vi "DFD FXP NStage MRate Modeling.vi"(4 "internal precision":T6, 5 "interstage word lengths":i16[](array[numeric]), 6 "output rounding mode":T4, 7 "input integer word length":i16=1, 8 "error in (no error)":errorcluster, 9 "output word length":i16=16, 10 "input word length":i16=16, 11 "multirate filters in":T1[](array[typedef]) {"mMRate_SumWl" min=1 max=32 step=1; "mMRate_InputIwl" min=1 max=32 step=1; "mMRate_GainWl" min=1 max=32 step=1; "mMRate_OutputWl" min=1 max=32 step=1; "mMRate_InputWl" min=1 max=32 step=1; "mMRate_CoefWl" min=1 max=32 step=1; "mMRate_Mode" items=["Default"=-1, "No Rate Change"=0, "Interpolation"=1, "Decimation"=2, "Interpolated"=3, "Rational"=4]}) -> (0 "error out":errorcluster, 3 "multirate filters out":T1[](array[typedef]) {"mMRate_SumWl" min=1 max=32 step=1; "mMRate_InputIwl" min=1 max=32 step=1; "mMRate_GainWl" min=1 max=32 step=1; "mMRate_OutputWl" min=1 max=32 step=1; "mMRate_InputWl" min=1 max=32 step=1; "mMRate_CoefWl" min=1 max=32 step=1; "mMRate_Mode" items=["Default"=-1, "No Rate Change"=0, "Interpolation"=1, "Decimation"=2, "Interpolated"=3, "Rational"=4]})   [LabVIEW 2017, in "NI_DigFilterLicensed.lvlib"]
doc: "Creates a fixed-point multistage multirate filter model according to the settings of the input word length, input integer word length, and output word length."
uses:
  <vilib>/addons/Digital Filter Design/NI_DigFilterLicensed.lvlib
  <vilib>/addons/Digital Filter Design/_Objects.llb/DFD FXP MRate Internal Precision Mode.ctl
  <vilib>/addons/Digital Filter Design/_Objects.llb/DFD Round-off Mode.ctl
  <vilib>/addons/Digital Filter Design/_Objects.llb/DFD Multirate Filter Obj.ctl
  <vilib>/addons/Digital Filter Design/_Objects.llb/DFD Multirate Mode.ctl
  <vilib>/addons/Digital Filter Design/_Objects.llb/DFD Coef Norm Type.ctl
  <vilib>/addons/Digital Filter Design/_Objects.llb/DFD FXP MRate Multiply Mode.ctl
  <vilib>/addons/Digital Filter Design/NI_DigFilter_FXP.lvlib
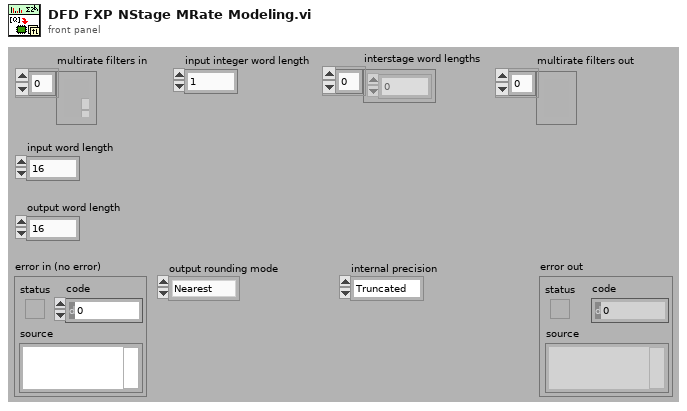
[diagram p1: front panel]
types:
  T1 = typedef "NI_DigFilterLicensed.lvlib/DFD Multirate Filter Obj.ctl" = cluster{"mMRate_Structure":enum16{"CIC", "FIR", "IIR", "Lattice"}, "mMRate_Mode":T2, "mMRate_Factor":i32, "mMRate_FIRParams":cluster{"mMRate_FIR_H":dbl[], "mMRate_FIR_IsNyquist?":bool, "mMRate_FIR_IsSymmetric?":bool}, "mMRate_CICParams":cluster{"mMRate_CIC_#Stage":i32, "mMRate_CIC_Lag":i32, "mMRate_CIC_Type":enum16{"Lowpass", "Highpass"}}, "mMRate_Order":i32, "mMRate_Version":string, "mMRate_Comments":string, "mMRate_RationalFactor":cluster{"mMRate_L":i32, "mMRate_M":i32}, "mMRate_Fs":dbl, "mMRate_Quantized?":bool, "mMRate_QFilterGain":dbl, "mMRate_CoefWl":i16, "mMRate_Scaling":cluster{"mMRate_ScaleByPowerOf2?":bool, "mMRate_ScaleType":T3}, "mMRate_InputWl":i16, "mMRate_OutputWl":i16, "mMRate_OutputMode":T4, "mMRate_MultMode":T5, "mMRate_BitPruning":bool, "mMRate_GainWl":i16, "mMRate_OutputFwl":i16, "mMRate_SumIwl":i16, "mMRate_InputIwl ":i16, "mMRate_SumWl":i16, "mMRate_CoefIwl":i16}
  T2 = typedef "NI_DigFilterLicensed.lvlib/DFD Multirate Mode.ctl" = i16
  T3 = typedef "NI_DigFilterLicensed.lvlib/DFD Coef Norm Type.ctl" = enum16{"No Norm", "Time Domain 1-Norm", "Time Domain 2-Norm", "Time Domain Inf-Norm"}
  T4 = typedef "NI_DigFilterLicensed.lvlib/DFD Round-off Mode.ctl" = enum16{"Nearest", "Truncation"}
  T5 = typedef "NI_DigFilterLicensed.lvlib/DFD FXP MRate Multiply Mode.ctl" = enum16{"Truncated", "Full"}
  T6 = typedef "NI_DigFilterLicensed.lvlib/DFD FXP MRate Internal Precision Mode.ctl" = enum16{"Truncated", "Full"}
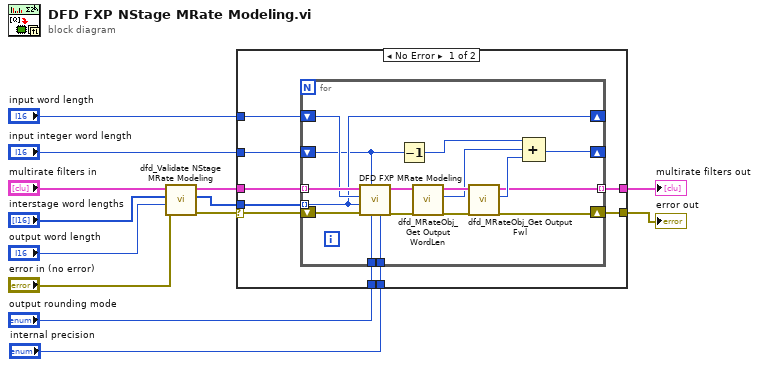
[diagram p0: block diagram]
diagram:
  n1 = call <vilib>:"dfd_Validate NStage MRate Modeling.vi"("error in (no error)"="error in (no error)", "output wl"="output word length", "interstage wl"="interstage word lengths", "multirate filters in"="multirate filters in") -> ("error out"=w2:errorcluster, "all-stage output wl"=w5:i16[], "dup multirate filters in"=w10:T1[])  [unwired: 5 out]
  n2 = case shown="No Error" w2 {
    selector: w2 -> [w15 w38]
    tunnel: [w22 _] -> w13
    tunnel: [w21 w38] -> w12
    tunnel: w10 -> [w20 _]
    tunnel: "input word length" -> [w19 _]
    tunnel: w5 -> [w18 _]
    tunnel: "output rounding mode" -> [w17 _]
    tunnel: "internal precision" -> [w16 _]
    tunnel: "input integer word length" -> [w14 _]
    frame No Error {
      n3 = for {
        tunnel: w20 -> [w37] mode=indexing
        shift-right: [w28] -> w21
        shift-left: w15 -> [w36]
        tunnel: w16 -> [w32]
        tunnel: w17 -> [w33]
        tunnel: [w29] -> w22 mode=indexing
        shift-right: [w34] -> _
        shift-left: w19 -> [w35]
        tunnel: w18 -> [w34] mode=indexing
        shift-right: [w31] -> _
        shift-left: w14 -> [w23]
        n4 = call <vilib>:"DFD FXP MRate Modeling.vi"("internal precision"=w32, "output rounding mode"=w33, "input integer word length"=w23, "error in (no error)"=w36, "output word length"=w34, "input word length"=w35, "multirate filter in"=w37) -> ("error out"=w28:errorcluster, "multirate filter out"=w27:T1)  [unwired: 1 in, 2 out]
        n5 = Decrement(x=w23) -> (x-1=w24:i16)
        n6 = call <vilib>:"dfd_MRateObj_Get Output WordLen.vi"("multirate filter in"=w27) -> ("output wl"=w25:i16, "dup multirate filter"=w26:T1)  [unwired: 9 out]
        n7 = call <vilib>:"dfd_MRateObj_Get Output Fwl.vi"("multirate filter in"=w26) -> ("output fwl"=w30:i16, "dup multirate filter"=w29:T1)  [unwired: 1 in, 8 out]
        n8 = Compound Arithmetic op=ADD(w24, w25, w30) -> (w31:i16)
      }
    }
    frame Error {
    }
  }
  "error out" <- w12
  "multirate filters out" <- w13
